vi "JKI-SM Example.vi"() -> ()   [LabVIEW 2013]
uses:
  <vilib>/LabVIEW Open Source Project/Cron Scheduler/Job/Job Report -- cluster.ctl
  <vilib>/LabVIEW Open Source Project/Cron Scheduler/Job/Job.lvclass/Job.ctl
  <vilib>/LabVIEW Open Source Project/Cron Scheduler/JobReport/JobReport.lvclass/JobReport.ctl
  <vilib>/LabVIEW Open Source Project/Cron Scheduler/Cron/Create Cron Expression.vi
  <vilib>/LabVIEW Open Source Project/Cron Scheduler/Cron/Compute Next Cron.vi
  <vilib>/LabVIEW Open Source Project/Cron Scheduler/Cron.Quartz/Cron.Quartz.lvclass
  <vilib>/LabVIEW Open Source Project/Cron Scheduler/Job/Job.lvclass
  <vilib>/LabVIEW Open Source Project/Cron Scheduler/openCron.lvlib
  <vilib>/LabVIEW Open Source Project/Cron Scheduler/JobReport/JobReport.lvclass
  <vilib>/LabVIEW Open Source Project/Cron Scheduler/Job.StaticVIRef/Job.StaticVIRef.lvclass
panel:
  out "start time":timestamp
  out "GUID":string
  out "Job Started":string
  out "last error":errorcluster
  in  "Kill Job":bool
  in  "Abort Job":bool
  out "Job Report":T1
  out "Map":variant
  in  "Cron Expression":string="0/10 * * ? * *"
  out "syntax valid?":bool
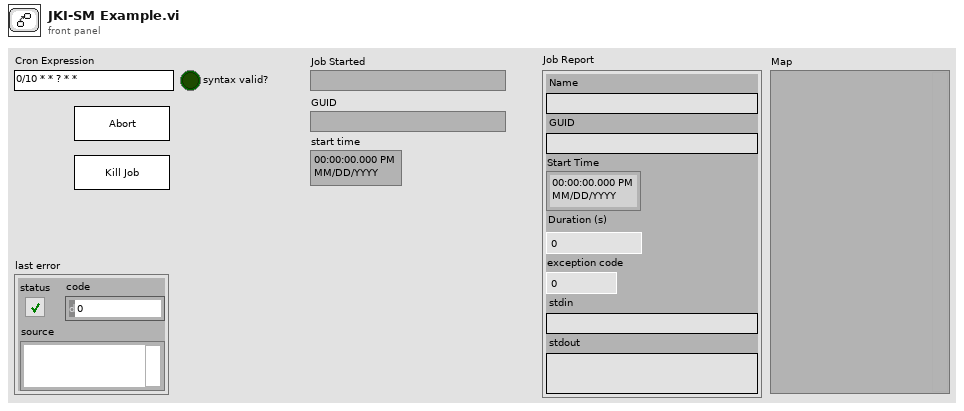
[diagram p1: front panel]
types:
  T1 = typedef "openCronJob.lvlib/JobReport.lvclass/Job Report -- cluster.ctl" = cluster{"Name":string, "GUID":string, "Start Time":timestamp, "Duration (s)":dbl, "exception code":i32, "stdin":string, "stdout":string}
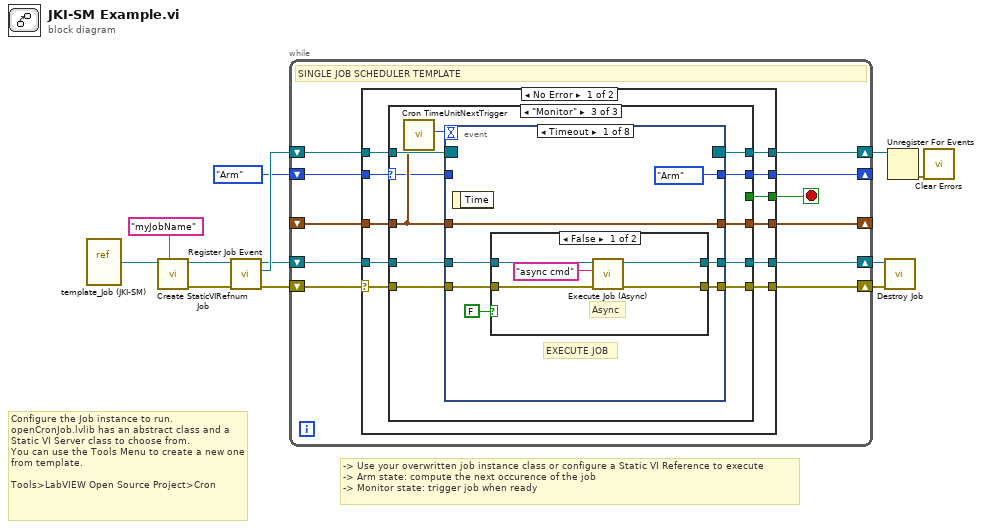
[diagram p0: block diagram]
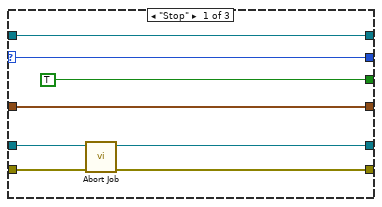
[diagram p2: hidden frame]
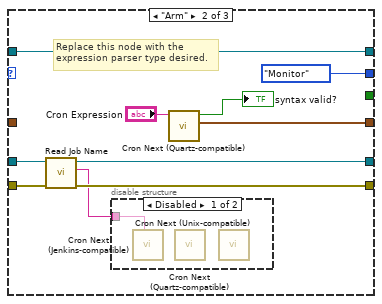
[diagram p3: hidden frame]
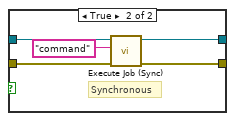
[diagram p5: hidden frame]
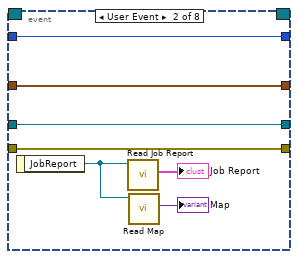
[diagram p6: hidden frame]
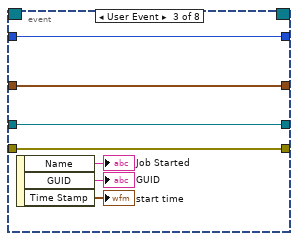
[diagram p7: hidden frame]
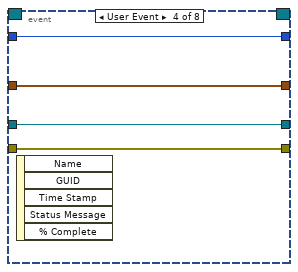
[diagram p8: hidden frame]
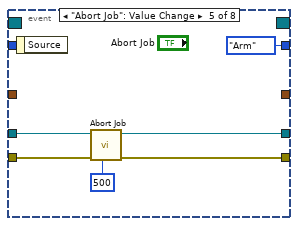
[diagram p9: hidden frame]
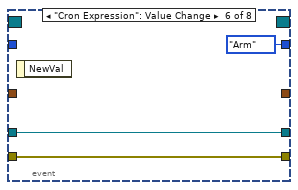
[diagram p10: hidden frame]
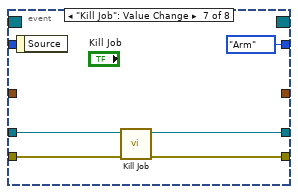
[diagram p11: hidden frame]
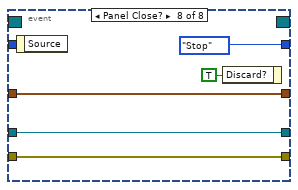
[diagram p12: hidden frame]
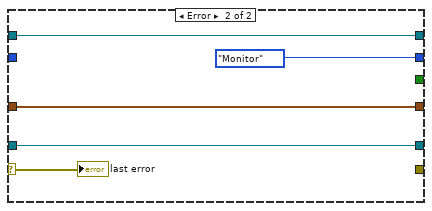
[diagram p13: hidden frame]
diagram:
  # "Configure the Job instance to run.\nopenCronJob.lvlib has an abstract class and a Static VI Server class to choose from.\nYou can use the Tools Menu to create a new one from template.\n\nTools>LabVIEW Open Source Project>Cron"
  # "-> Use your overwritten job instance class or configure a Static VI Reference to execute\n-> Arm state: compute the next occurence of the job\n-> Monitor state: trigger job when ready"
  n1 = vi-ref "template_Job (JKI-SM).vi"() -> (w11:refnum<vi>)
  n2 = call <vilib>:"Create StaticVIRefnum Job.vi"("Job Name"="myJobName", "Static VI Refnum"=w11) -> ("error out"=w7:errorcluster, "Job.StaticVIRef out"=w5:refnum<class "Job.StaticVIRef.lvclass">)  [unwired: 8 in]
  n3 = call <vilib>:"Register Job Event.vi"("Job in"=w5) -> ("Job Event Registration"=w9:refnum<event-registration>, "Job out"=w6:refnum<class "Job.StaticVIRef.lvclass">)  [unwired: 9 in]
  n4 = while {
    shift-right: [w21] -> _
    shift-left: _ -> [w22]
    shift-right: [w19] -> _
    shift-left: enum16{"Arm", "Stop", "Monitor"}."Arm" -> [w20]
    shift-right: [w16] -> w2
    shift-left: w9 -> [w17]
    shift-right: [w14] -> w4
    shift-left: w6 -> [w15]
    shift-right: [w13] -> w8
    shift-left: w7 -> [w12]
    stop <- w18 stop-if-true
    # "SINGLE JOB SCHEDULER TEMPLATE"
    n5 = case shown="No Error" w12 {
      selector: w12 -> [w23 w118]
      tunnel: w22 -> [w33 w120]
      tunnel: [w32 w120] -> w21
      tunnel: w20 -> [w31 _]
      tunnel: [w30 enum16{"Arm", "Stop", "Monitor"}."Monitor"] -> w19
      tunnel: [w29 _] -> w18
      tunnel: w17 -> [w28 w122]
      tunnel: [w27 w122] -> w16
      tunnel: w15 -> [w26 w119]
      tunnel: [w25 w119] -> w14
      tunnel: [w24 _] -> w13
      frame No Error {
        n6 = case shown="\"Monitor\"" w31 {
          selector: w31 -> [w41 _ w55]
          tunnel: w33 -> [w39 _ w58]
          tunnel: [w39 w50 w60] -> w32
          tunnel: [w41 enum16{"Arm", "Stop", "Monitor"}."Monitor" w61] -> w30
          tunnel: [TRUE _ _] -> w29
          tunnel: w28 -> [w38 w51 w63]
          tunnel: [w38 w51 w62] -> w27
          tunnel: w26 -> [w37 w44 w57]
          tunnel: [w36 w43 w56] -> w25
          tunnel: w23 -> [w35 w46 w54]
          tunnel: [w34 w45 w53] -> w24
          frame "Stop" {
            n7 = call <vilib>:"Abort Job.vi"("error in (no error)"=w35, "Job in"=w37) -> ("error out"=w34:errorcluster, "Job out"=w36:refnum<class "Job.StaticVIRef.lvclass">)  [unwired: 5 in, 3 out]
          }
          frame "Arm" {
            # "Replace this node with the\nexpression parser type desired."
            n8 = call <vilib>:"Read Job Name.vi"("error in (no error)"=w46, "Job in"=w44) -> ("error out"=w45:errorcluster, "Name"=w42:string, "Job out"=w43:refnum<class "Job.StaticVIRef.lvclass">)  [unwired: 7 in]
            n9 = disable-structure shown="Disabled" {
              disable-tunnel: w42 -> [w52 _]
              frame Disabled {
                n10 = call <vilib>:"Cron Next (Jenkins-compatible).vi"("Job Name"=w52) -> ()  [unwired: 8 in, 3 out]
                n11 = call <vilib>:"Cron Next (Quartz-compatible).vi"() -> ()  [unwired: 9 in, 3 out]
                n12 = call <vilib>:"Cron Next (Unix-compatible).vi"() -> ()  [unwired: 9 in, 3 out]
              }
              frame Enabled {
              }
            }
            n13 = call <vilib>:"Cron Next (Quartz-compatible).vi"("Cron Expression"="Cron Expression") -> ("Next Occurence"=w50:timestamp, "syntax valid?"=→"syntax valid?":bool)  [unwired: 8 in, 1 out]
          }
          frame "Monitor" {
            n14 = call <vilib>:"Cron TimeUnitNextTrigger.vi"("Next Occurence"=w58) -> ("next event (ms)"=w59:i32)  [unwired: 10 in]
            n15 = event shown="[0] Timeout" {
              selector: w63 -> [_ _ _ _ _ _ _ _]
              dyn-events: [_ _ _ _ _ _ _ _] -> w62
              timeout: w59 -> [_ _ _ _ _ _ _ _]
              tunnel: [enum16{"Arm", "Stop", "Monitor"}."Arm" w86 w93 w97 enum16{"Arm", "Stop", "Monitor"}."Arm" enum16{"Arm", "Stop", "Monitor"}."Arm" enum16{"Arm", "Stop", "Monitor"}."Arm" enum16{"Arm", "Stop", "Monitor"}."Stop"] -> w61
              tunnel: [w64 w87 w94 w98 _ _ _ w115] -> w60
              tunnel: w58 -> [w64 w87 w94 w98 _ _ _ w115]
              tunnel: w57 -> [w69 w85 w92 w96 w103 w106 w111 w114]
              tunnel: [w67 w85 w92 w96 w102 w106 w110 w114] -> w56
              tunnel: w55 -> [_ w86 w93 w97 _ _ _ _]
              tunnel: w54 -> [w66 w84 w91 w95 w100 w105 w109 w113]
              tunnel: [w65 w84 w91 w95 w99 w105 w108 w113] -> w53
              event Timeout {
                # "EXECUTE JOB"
                n16 = event-data() -> ()  [unwired: 1 in, 1 out]
                n17 = case shown="False" FALSE ("Synchronous?") {
                  tunnel: w69 -> [w75 w80]
                  tunnel: [w74 w79] -> w67
                  tunnel: w66 -> [w72 w78]
                  tunnel: [w73 w77] -> w65
                  frame False {
                    # "Async"
                    n18 = call <vilib>:"Execute Job (Async).vi"("error in (no error)"=w72, "stdin"="async cmd", "Job in"=w75) -> ("error out"=w73:errorcluster, "Job out"=w74:refnum<class "Job.StaticVIRef.lvclass">)  [unwired: 6 in, 1 out]
                  }
                  frame True {
                    # "Synchronous"
                    n19 = call <vilib>:"Execute Job (Sync).vi"("error in (no error)"=w78, "stdin"="command", "Job in"=w80) -> ("error out"=w77:errorcluster, "Job out"=w79:refnum<class "Job.StaticVIRef.lvclass">)  [unwired: 5 in, 2 out]
                  }
                }
              }
              event User Event {
                n20 = event-data() -> ("JobReport"=w82:refnum<class "JobReport.lvclass">)  [unwired: 1 in]
                n21 = call <vilib>:"Read Job Report.vi"("JobReport in"=w82) -> ("Job Report"=→"Job Report":T1)  [unwired: 8 in, 2 out]
                n22 = call <vilib>:"Read Map.vi"("JobReport in"=w82) -> ("Map"=→"Map":variant)  [unwired: 8 in, 2 out]
              }
              event User Event {
                n23 = event-data() -> ("Name"=→"Job Started":string, "GUID"=→"GUID":string, "Time Stamp"=→"start time":timestamp)  [unwired: 1 in]
              }
              event User Event {
                n24 = event-data() -> ()  [unwired: 1 in, 5 out]
              }
              event "Abort Job": Value Change {
                n25 = event-data() -> ()  [unwired: 1 in, 1 out]
                n26 = call <vilib>:"Abort Job.vi"("timeout (500 ms)"=500, "error in (no error)"=w100, "Job in"=w103) -> ("error out"=w99:errorcluster, "Job out"=w102:refnum<class "Job.StaticVIRef.lvclass">)  [unwired: 4 in, 3 out]
              }
              event "Cron Expression": Value Change {
                n27 = event-data() -> ()  [unwired: 1 in, 1 out]
              }
              event "Kill Job": Value Change {
                n28 = event-data() -> ()  [unwired: 1 in, 1 out]
                n29 = call <vilib>:"Kill Job.vi"("error in (no error)"=w109, "Job in"=w111) -> ("error out"=w108:errorcluster, "Job out"=w110:refnum<class "Job.StaticVIRef.lvclass">)  [unwired: 8 in]
              }
              event Panel Close? {
                n30 = event-data() -> ()  [unwired: 1 in, 1 out]
                n31 = event-data("Discard?"=TRUE) -> ()  [unwired: 1 in, 1 out]
              }
            }
          }
        }
      }
      frame Error {
        "last error" <- w118
      }
    }
  }
  n32 = call <vilib>:"Destroy Job.vi"("error in (no error)"=w8, "Job in"=w4) -> ()  [unwired: 8 in, 2 out]
  n33 = Unregister For Events(event registration refnum=w2) -> (error out=w3:errorcluster)  [unwired: 1 in]
  n34 = call <vilib>:"Clear Errors.vi"("error in (no error)"=w3) -> ()  [unwired: 6 in, 1 out]
